vi "Read Network Path.vi"(8 "error in (no error)":errorcluster, 10 "T/Y":bool, 11 "Base Path":path) -> (0 "error out":errorcluster, 2 "file or folder exists?":bool, 3 "appended path":path)   [LabVIEW 2014]
panel:
  # "Z:\\ST30\\Jun-2020\\Jun-10-20.xls"
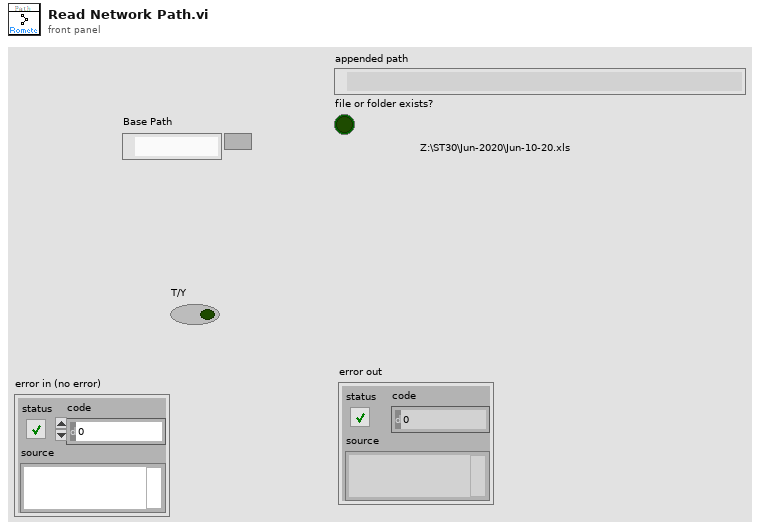
[diagram p1: front panel]
types:
  T1 = typedef "LVDateTimeRec.ctl" = cluster{"fractional second":dbl, "second":i32, "minute":i32, "hour":i32, "day of month":i32, "month":i32, "year":i32, "day of week":i32, "day of year":i32, "DST":i32}
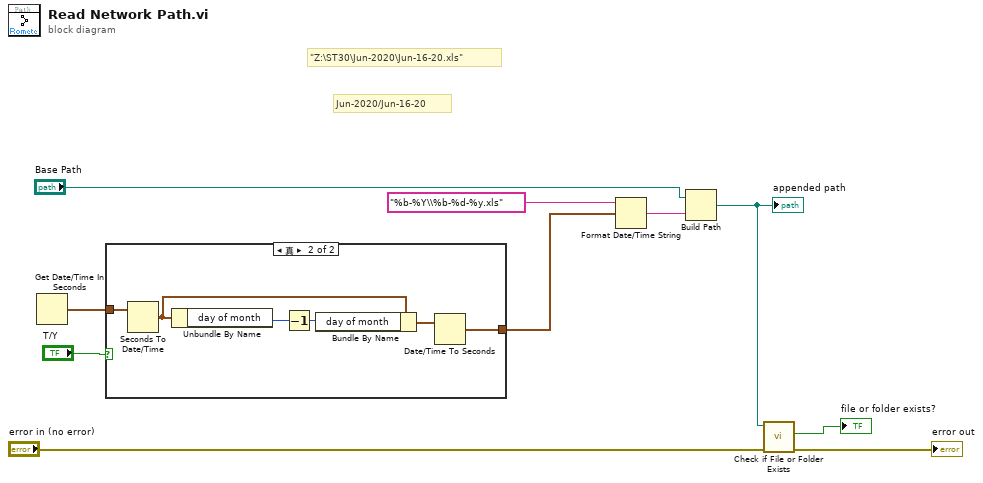
[diagram p0: block diagram]
diagram:
  # "Jun-2020/Jun-16-20"
  # "\"Z:\\ST30\\Jun-2020\\Jun-16-20.xls\""
  n1 = Get Date/Time In Seconds() -> (seconds since 1Jan1904=w9:timestamp)
  n2 = case shown="真" "T/Y" {
    tunnel: w9 -> [w11 w14]
    tunnel: [w11 w12] -> w8
    frame False {
    }
    frame True {
      n3 = Seconds To Date/Time(time stamp (now)=w14) -> (date time rec=w13:T1)  [unwired: 1 in]
      n4 = Unbundle By Name(w13) -> ("day of month"=w17:i32)
      n5 = Decrement(x=w17) -> (x-1=w16:i32)
      n6 = Bundle By Name(cluster=w13, "day of month"=w16) -> (w15:T1)
      n7 = Date/Time To Seconds(2:w15) -> (0:w12:timestamp)  [unwired: 1 in]
    }
  }
  n8 = Format Date/Time String(time format string (%c)="%b-%Y\\%b-%d-%y.xls", seconds (now)=w8) -> (date/time string=w6:string)  [unwired: 1 in]
  n9 = Build Path(base path="Base Path", name or relative path=w6) -> (appended path=w3:path)
  "appended path" <- w3
  n10 = call <vilib>:"Check if File or Folder Exists.vi"("error in (no error)"="error in (no error)", "path"=w3) -> ("error out"=→"error out":errorcluster, "file or folder exists?"=→"file or folder exists?":bool)  [unwired: 7 in, 1 out]
